vi "Send Software Trigger Core.vi"(8 "error in (no error)":errorcluster, 11 "CS++DMM in":refnum<class "CS++DMM.lvclass">) -> (0 "error out":errorcluster, 3 "CS++DMM out":refnum<class "CS++DMM.lvclass">)   [LabVIEW 2013, in "CS++DMM.lvlib" / "CS++DMM.lvclass"]
doc: "This VI sends a command to trigger the DMM. Call this VI if you pass IVIDMM_VAL_SOFTWARE_TRIG for the Trigger Source parameter of the Configure Trigger VI or the Sample Trigger parameter of the Configure Multi-Point [MP] VI.\n\nNotes:\n\n(1) This VI is part of the IviDmmSoftwareTrigger [SWT] extension group.\n\n(2) If neither the IviDmm>Trigger>Trigger Source nor the IviDmm>Multi-Point Acquisition>Sample Trigger [MP] property is set to the IVIDMM_VAL_SOFTWARE_TRIG value, this VI returns an error.\n\n(3) This VI does not check the instrument status. Typically, you call this VI only in a sequence of calls to other low-level driver VIs. The sequence performs one operation. You use the low-level VIs to optimize one or more aspects of interaction with the instrument. If you want to check the instrument status, call the Error-Query VI at the conclusion of the sequence."
uses:
  CS++DMM.lvclass
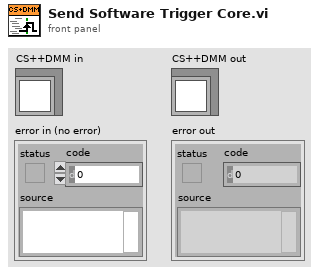
[diagram p1: front panel]
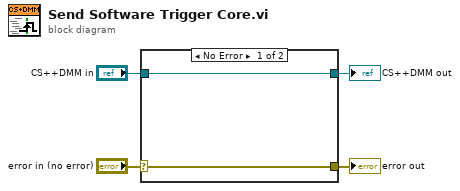
[diagram p0: block diagram]
diagram:
  n1 = case shown="No Error" "error in (no error)" {
    selector: "error in (no error)" -> [w5 w8]
    tunnel: [w5 w8] -> w3
    tunnel: [w6 w7] -> w1
    tunnel: "CS++DMM in" -> [w6 w7]
    frame No Error {
    }
    frame Error {
    }
  }
  "error out" <- w3
  "CS++DMM out" <- w1
